vi "Check for Target Crossing.vi"(6 "output power":dbl, 7 "first call?":bool, 8 "error in (no error)":errorcluster, 9 "previous measured value":dbl, 10 "results":T15, 11 "measurement configuration":T1 {"acq sampling rate" format="%0.2f"; "master clock rate" format="%#_6pHz"; "frame clock rate" format="%#_6pHz"}) -> (0 "error out":errorcluster, 1 "measured value":dbl, 3 "crossing found?":bool)   [LabVIEW 2021, in "Stepped Frequency Sweep_Class D Amplifier.lvlib"]
uses:
  Stepped Frequency Sweep_Class D Amplifier.lvlib
  shared/controls/single tone audio measurements.ctl
  Measurement Configuration.ctl
  shared/controls/digital audio protocol/data justification.ctl
  shared/controls/digital audio protocol/endianness.ctl
  shared/controls/digital audio protocol/digital edge.ctl
  shared/controls/digital audio protocol/logic level.ctl
  shared/controls/digital output level units.ctl
  shared/controls/weighting filter.ctl
  shared/controls/highpass filter.ctl
  shared/controls/lowpass filter.ctl
  shared/controls/sweep profile.ctl
  shared/controls/units - snr.ctl
  shared/controls/units - ratio.ctl
  shared/controls/regulation target.ctl
  shared/controls/regulation target value units.ctl
  shared/controls/audio controls.lvlib
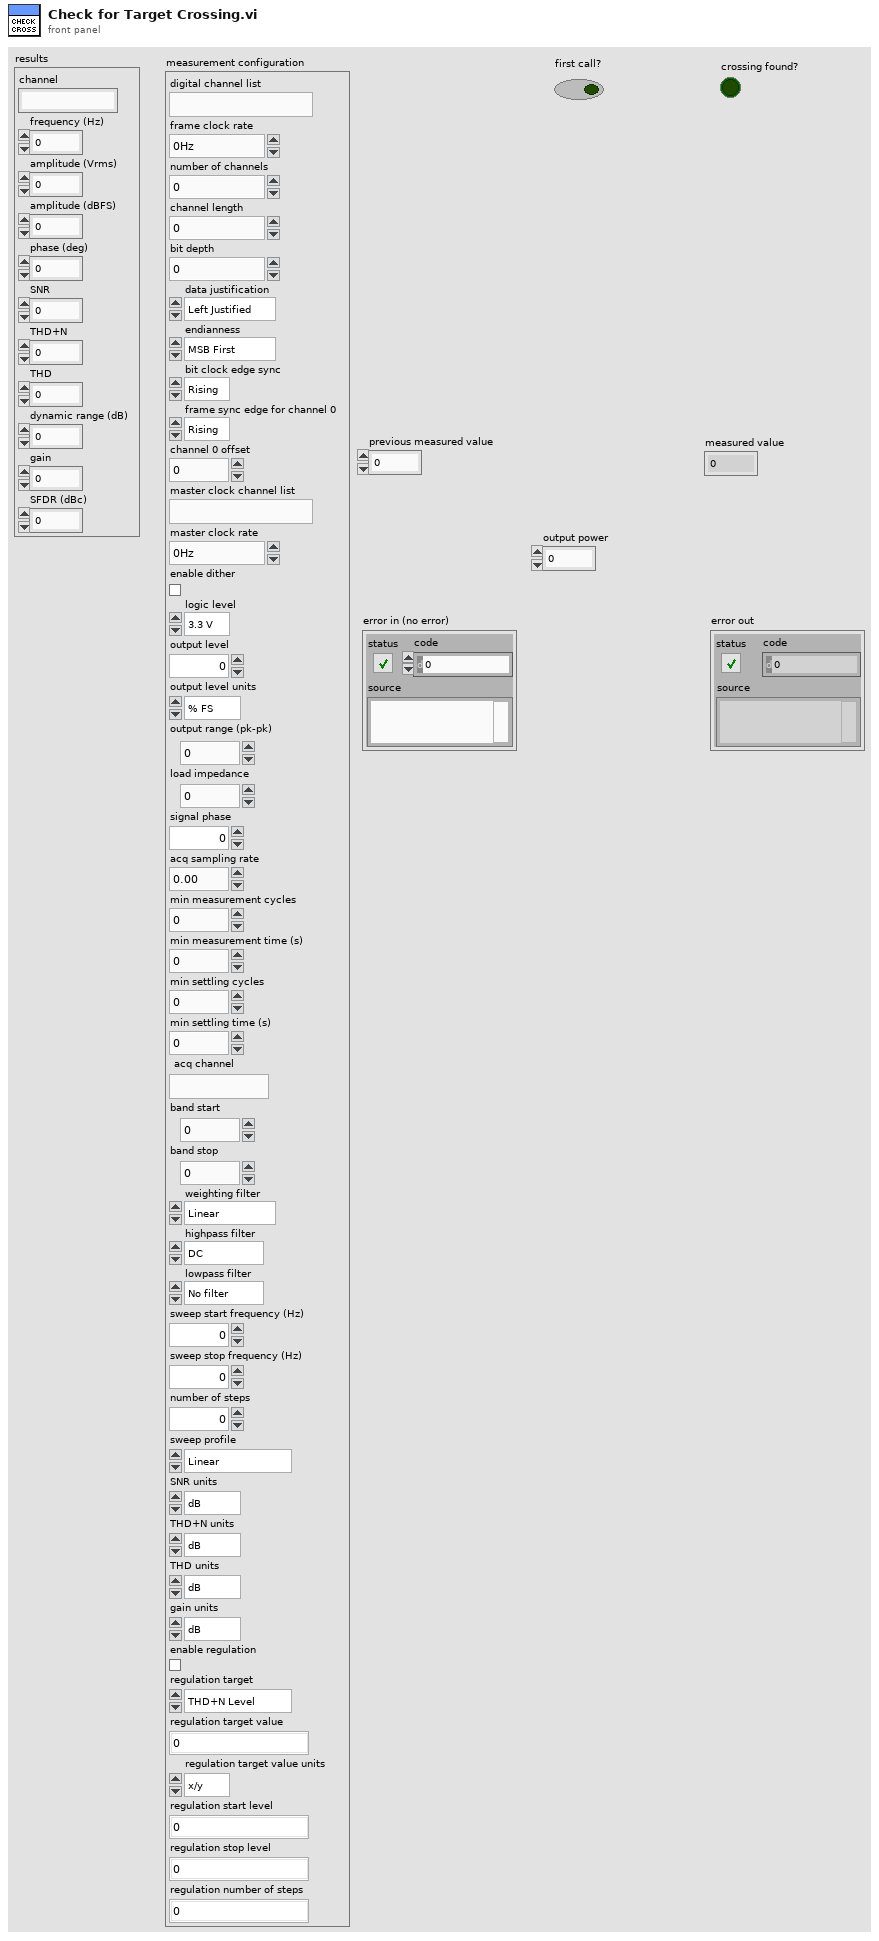
[diagram p1: front panel]
types:
  T1 = typedef "Stepped Frequency Sweep_Class D Amplifier.lvlib/Measurement Configuration.ctl" = cluster{"digital channel list":string, "frame clock rate":dbl, "number of channels":u32, "channel length":u32, "bit depth":u32, "data justification":T2, "endianness":T3, "bit clock edge sync":T4, "frame sync edge for channel 0":T4, "channel 0 offset":u32, "master clock channel list":string, "master clock rate":dbl, "enable dither":bool, "logic level":T5, "output level":dbl, "output level units":T6, "output range (pk-pk)":dbl, "load impedance":dbl, "signal phase":dbl, "acq sampling rate":dbl, "min measurement cycles":u32, "min measurement time (s)":dbl, "min settling cycles":u32, "min settling time (s)":dbl, "acq channel":string, "band start":dbl, "band stop":dbl, "weighting filter":T7, "highpass filter":T8, "lowpass filter":T9, "sweep start frequency (Hz)":dbl, "sweep stop frequency (Hz)":dbl, "number of steps":u32, "sweep profile":T10, "SNR units":T11, "THD+N units":T12, "THD units":T12, "gain units":T12, "enable regulation":bool, "regulation target":T13, "regulation target value":dbl, "regulation target value units":T14, "regulation start level":dbl, "regulation stop level":dbl, "regulation number of steps":u32}
  T2 = typedef "data justification.ctl" = enum32{"Left Justified", "Right Justified"}
  T3 = typedef "endianness.ctl" = enum32{"MSB First", "LSB First"}
  T4 = typedef "digital edge.ctl" = enum32{"Rising", "Falling"}
  T5 = typedef "logic level.ctl" = enum32{"3.3 V", "1.8 V", "1.2 V"}
  T6 = typedef "audio controls.lvlib/digital output level units.ctl" = enum32{"% FS", "dBFS"}
  T7 = typedef "weighting filter.ctl" = enum32{"Linear", "A-weighting", "B-weighting", "C-weighting"}
  T8 = typedef "highpass filter.ctl" = enum32{"DC", "AC"}
  T9 = typedef "lowpass filter.ctl" = enum32{"No filter", "AES17 20kHz", "AES17 40kHz"}
  T10 = typedef "audio controls.lvlib/sweep profile.ctl" = enum32{"Linear", "Logarithmic"}
  T11 = typedef "audio controls.lvlib/units - snr.ctl" = enum32{"dB", "x/y"}
  T12 = typedef "audio controls.lvlib/units - ratio.ctl" = enum32{"dB", "%", "x/y"}
  T13 = typedef "regulation target.ctl" = enum32{"THD+N Level", "THD+N Ratio", "RMS Level", "RMS Ratio", "Output Power"}
  T14 = typedef "regulation target value units.ctl" = enum32{"x/y", "%", "dB", "Vrms", "W"}
  T15 = typedef "audio controls.lvlib/single tone audio measurements.ctl" = cluster{"channel":string, "frequency (Hz)":dbl, "amplitude (Vrms)":dbl, "amplitude (dBFS)":dbl, "phase (deg)":dbl, "SNR":dbl, "THD+N":dbl, "THD":dbl, "dynamic range (dB)":dbl, "gain":dbl, "SFDR (dBc)":dbl}
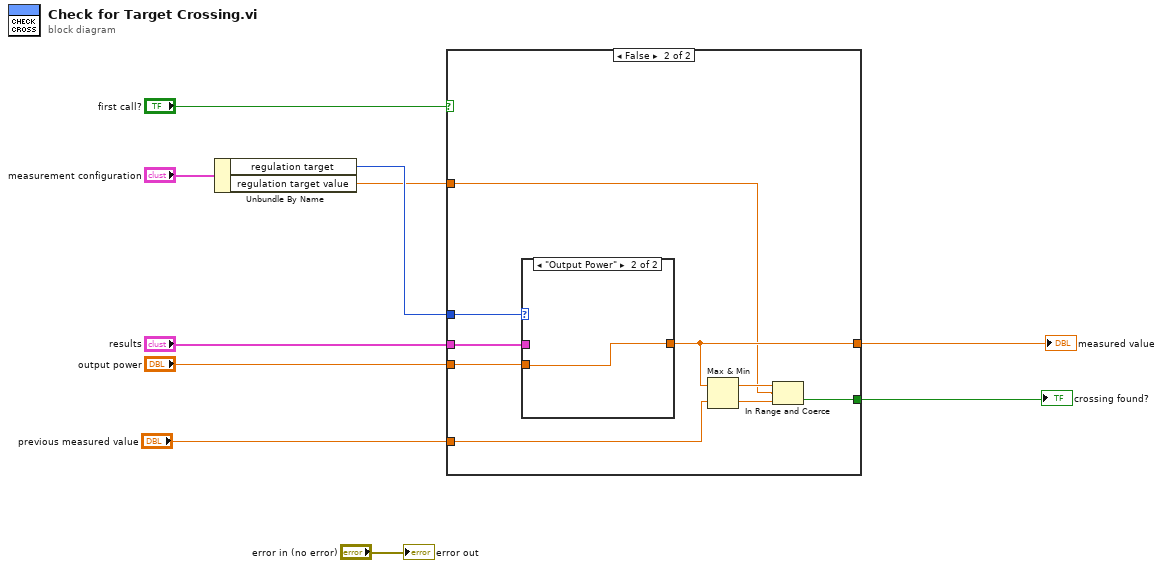
[diagram p0: block diagram]
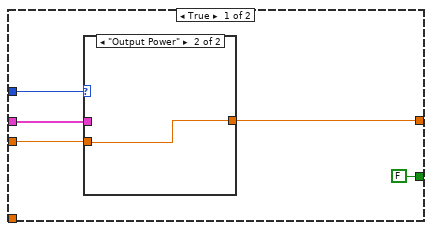
[diagram p2: hidden frame]
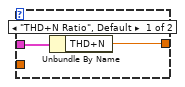
[diagram p3: hidden frame]
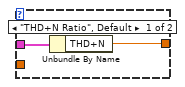
[diagram p4: hidden frame]
diagram:
  n1 = Unbundle By Name("measurement configuration") -> ("regulation target"=w7:T13, "regulation target value"=w2:dbl)
  n2 = case shown="False" "first call?" {
    tunnel: "results" -> [w15 w27]
    tunnel: w7 -> [w14 w26]
    tunnel: "output power" -> [w13 w25]
    tunnel: [w12 w23] -> w5
    tunnel: "previous measured value" -> [_ w24]
    tunnel: w2 -> [_ w20]
    tunnel: [FALSE w19] -> w1
    frame True {
      n3 = case shown="\"Output Power\"" w14 {
        tunnel: w15 -> [w17 _]
        tunnel: [w16 w18] -> w12
        tunnel: w13 -> [_ w18]
        frame "THD+N Ratio", Default {
          n4 = Unbundle By Name(w17) -> ("THD+N"=w16:dbl)
        }
        frame "Output Power" {
        }
      }
    }
    frame False {
      n5 = case shown="\"Output Power\"" w26 {
        tunnel: w27 -> [w29 _]
        tunnel: [w28 w30] -> w23
        tunnel: w25 -> [_ w30]
        frame "THD+N Ratio", Default {
          n6 = Unbundle By Name(w29) -> ("THD+N"=w28:dbl)
        }
        frame "Output Power" {
        }
      }
      n7 = Max & Min(x=w23, y=w24) -> (max(x,y)=w22:dbl, min(x,y)=w21:dbl)
      n8 = In Range and Coerce(upper limit=w22, x=w20, lower limit=w21) -> (In Range?=w19:bool)  [unwired: 1 out]
    }
  }
  "crossing found?" <- w1
  "measured value" <- w5
  "error out" <- "error in (no error)"
